vi "Set Locale Settings.vi"(9 "Locale":string, 10 "Decimal":T1, 11 "MsgSerializer":refnum<class "MsgSerializer.lvclass">) -> (3 "MsgSerializer":refnum<class "MsgSerializer.lvclass">)   [LabVIEW 2013, in "Caraya.lvlib" / "MsgSerializer.lvclass"]
uses:
  MsgSerializer/MsgSerializer.lvclass
  decimal-notation -- enum.ctl
  MsgSerializer/MsgSerializer.lvclass/MsgSerializer.ctl
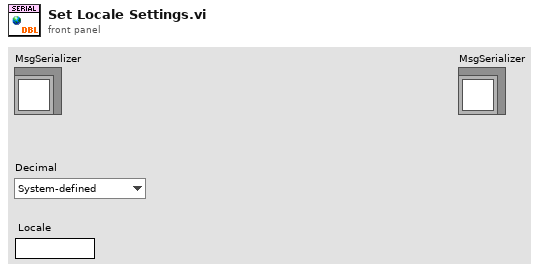
[diagram p1: front panel]
types:
  T1 = typedef "Caraya.lvlib/MsgSerializer.lvclass/decimal-notation -- enum.ctl" = enum16{"System-defined", "dot-notation", "comma-notation"}
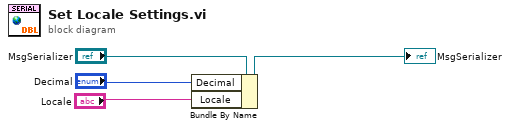
[diagram p0: block diagram]
diagram:
  n1 = Bundle By Name(cluster="MsgSerializer", "Decimal"="Decimal", "Locale"="Locale") -> (→"MsgSerializer":refnum<class "MsgSerializer.lvclass">)
